vi "Analyze reward conditions - No VR.vi"(6 "Lick event":bool, 7 "Array":i32[](array[numeric]), 9 "reward given":u32, 10 "mouse position":dbl) -> (1 "Active rew within RZ":bool, 2 "Passive rew within RZ":bool, 4 "Passive rew after RZ":bool, 5 "Within reward zone":bool)   [LabVIEW 2017]
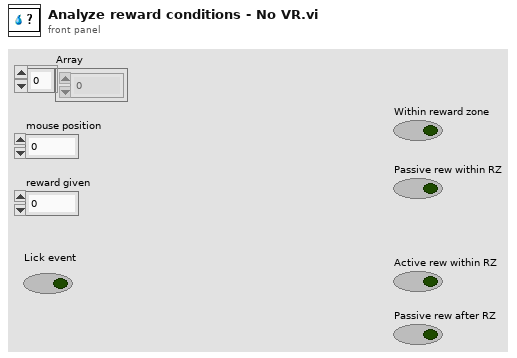
[diagram p1: front panel]
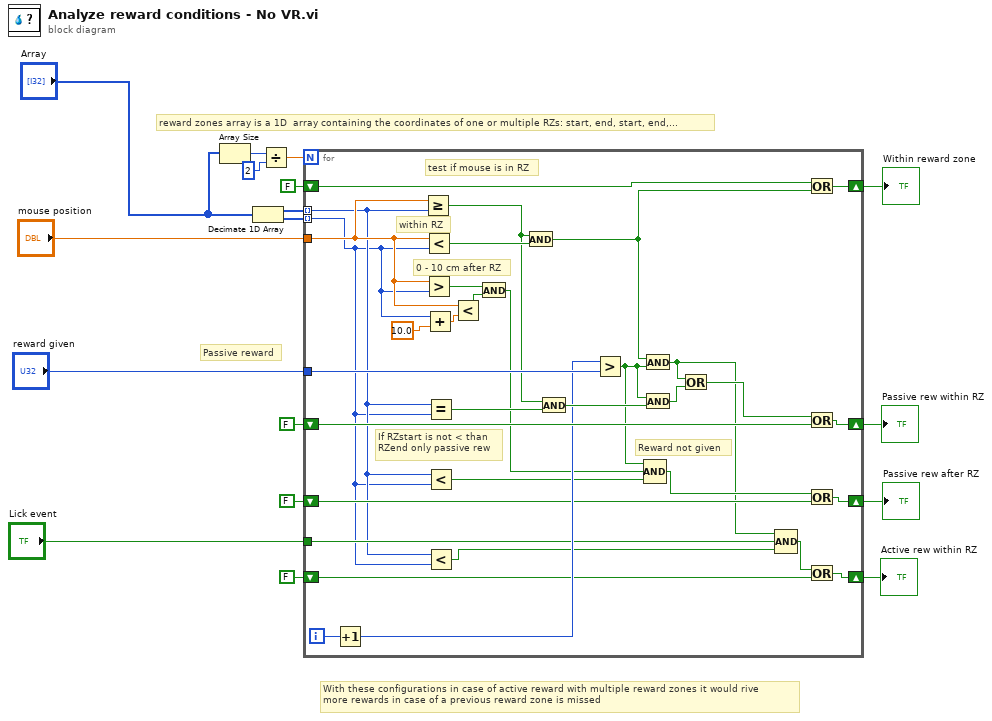
[diagram p0: block diagram]
diagram:
  # "With these configurations in case of active reward with multiple reward zones it would rive\nmore rewards in case of a previous reward zone is missed"
  # "Passive reward"
  # "reward zones array is a 1D  array containing the coordinates of one or multiple RZs: start, end, start, end,..."
  n1 = Array Size(array="Array") -> (size(s)=w13:i32)
  n2 = Decimate 1D Array("Array") -> (w6:i32[], w7:i32[])
  n3 = Divide(x=w13, y=2) -> (x/y=w14:dbl)
  n4 = for {
    N: w14 -> [_]
    tunnel: w6 -> [w21] mode=indexing
    tunnel: w7 -> [w20] mode=indexing
    tunnel: "mouse position" -> [w35]
    shift-right: [w48] -> w10
    shift-left: FALSE -> [w39]
    tunnel: "reward given" -> [w49]
    shift-right: [w42] -> w16
    shift-left: FALSE -> [w43]
    shift-right: [w32] -> w5
    shift-left: FALSE -> [w28]
    shift-right: [w27] -> w3
    shift-left: FALSE -> [w26]
    tunnel: "Lick event" -> [w23]
    i -> [w41]
    # "If RZstart is not < than \nRZend only passive rew"
    # "test if mouse is in RZ"
    # "0 - 10 cm after RZ"
    # "within RZ"
    # "Reward not given"
    n5 = Increment(x=w41) -> (x+1=w40:i32)
    n6 = Greater Or Equal?(x=w35, y=w21) -> (x >= y?=w47:bool)
    n7 = Less?(x=w35, y=w20) -> (x < y?=w50:bool)
    n8 = Greater?(x=w35, y=w20) -> (0:w33:bool)
    n9 = Add(x=w20, y=10.0) -> (x+y=w37:dbl)
    n10 = Equal?(x=w21, y=w20) -> (x = y?=w46:bool)
    n11 = Less?(x=w21, y=w20) -> (x < y?=w19:bool)
    n12 = Less?(x=w21, y=w20) -> (x < y?=w18:bool)
    n13 = Less?(x=w35, y=w37) -> (x < y?=w34:bool)
    n14 = And(x=w33, y=w34) -> (x .and. y?=w30:bool)
    n15 = And(x=w47, y=w50) -> (x .and. y?=w38:bool)
    n16 = And(x=w47, y=w46) -> (x .and. y?=w45:bool)
    n17 = Greater?(x=w40, y=w49) -> (0:w29:bool)
    n18 = And(x=w38, y=w29) -> (x .and. y?=w24:bool)
    n19 = And(x=w29, y=w45) -> (x .and. y?=w44:bool)
    n20 = Compound Arithmetic op=AND(w29, w30, w19) -> (w31:bool)
    n21 = Or(x=w24, y=w44) -> (x .or. y?=w25:bool)
    n22 = Compound Arithmetic op=AND(w24, w23, w18) -> (w22:bool)
    n23 = Or(x=w39, y=w38) -> (x .or. y?=w48:bool)
    n24 = Or(x=w25, y=w43) -> (x .or. y?=w42:bool)
    n25 = Or(x=w31, y=w28) -> (x .or. y?=w32:bool)
    n26 = Or(x=w22, y=w26) -> (x .or. y?=w27:bool)
  }
  "Passive rew within RZ" <- w16
  "Within reward zone" <- w10
  "Passive rew after RZ" <- w5
  "Active rew within RZ" <- w3
